vi "菜单-编译.vi"(8 "error in (no error)":errorcluster caption="错误输入（无错误）", 11 "程序响应 输入":refnum<class "程序响应.lvclass">) -> (0 "error out":errorcluster caption="错误输出", 3 "程序响应 输出":refnum<class "程序响应.lvclass">)   [LabVIEW 2020, in "程序响应.lvlib" / "程序响应.lvclass"]
uses:
  D:/SuperPython-master/ScintillaNET.dll
  ScintillaNET.dll
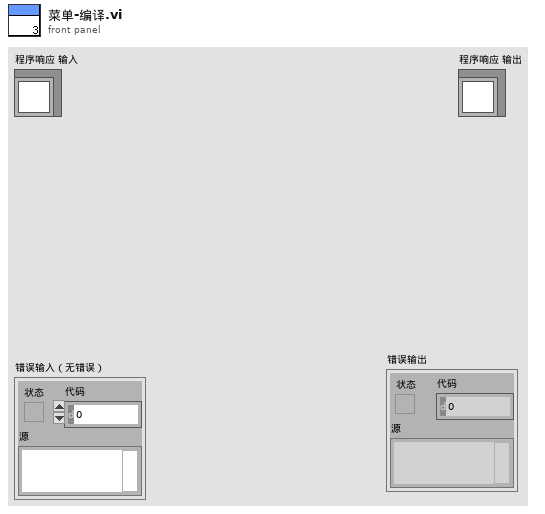
[diagram p1: front panel]
types:
  T1 = enum16{"open", "replace", "create", "open or create", "replace or create", "replace or create with confirmation"}
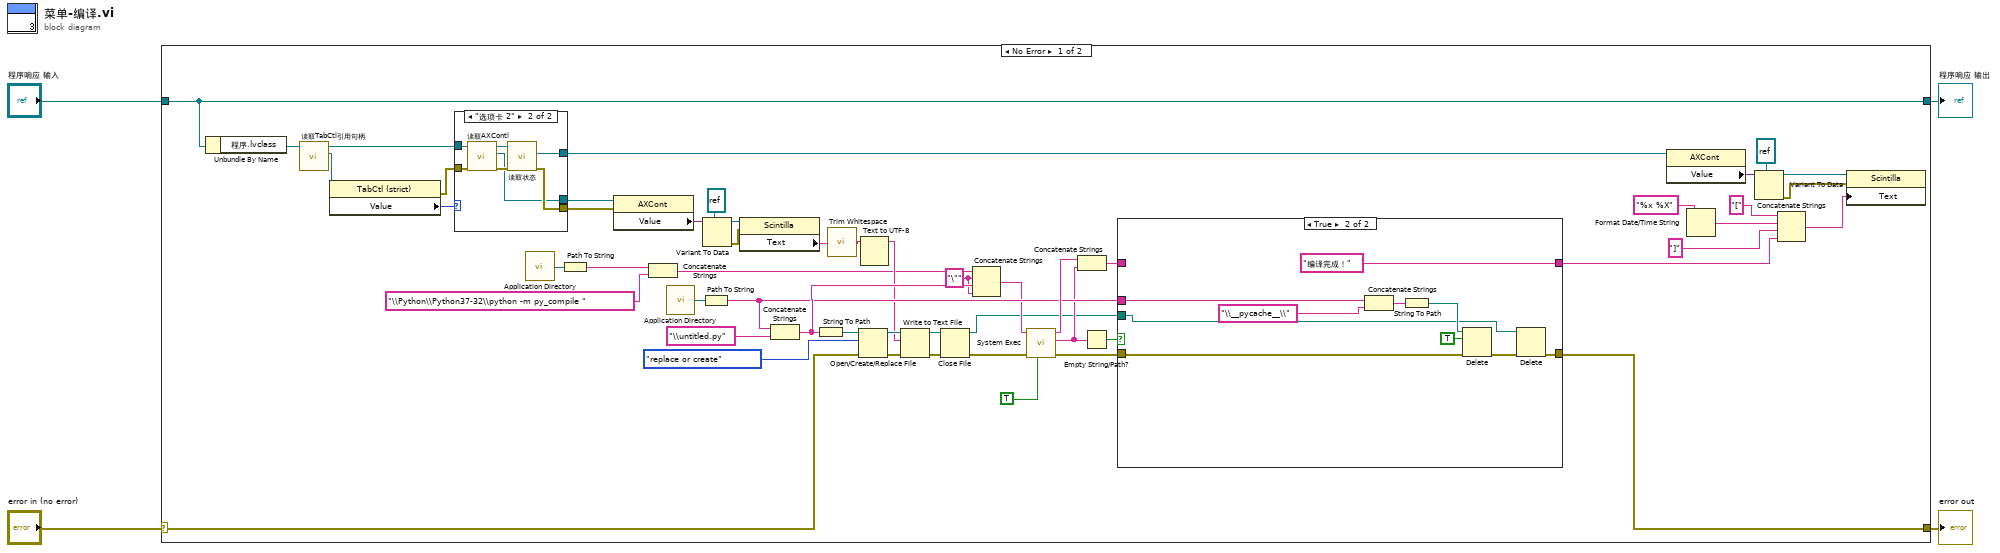
[diagram p0: block diagram]
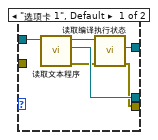
[diagram p2: hidden frame]
diagram:
  n1 = case shown="No Error" "error in (no error)" {
    selector: "error in (no error)" -> [w42 w83]
    tunnel: [w41 w83] -> w3
    tunnel: [w44 w82] -> w1
    tunnel: "程序响应 输入" -> [w44 w82]
    frame No Error {
      w11 = "\"" ("字符串")
      n2 = Unbundle By Name(w44) -> ("程序.lvclass"=w16:refnum<class "程序.lvclass">)
      n3 = call-dynamic "读取TabCtl引用句柄.vi"("程序输入"=w16) -> ("TabCtl引用句柄"=w15:refnum<vi>, "程序输出"=w12:refnum<class "程序.lvclass">)  [unwired: 8 in, 1 out]
      n4 = property class="TabCtl (strict)"(reference=w15) -> (error out=w13:errorcluster, "Value"=w14:enum32{"选项卡 1", "选项卡 2"})  [unwired: 1 in, 1 out]
      n5 = case shown="\"选项卡 2\"" w14 {
        tunnel: [w61 w63] -> w25
        tunnel: [w57 w64] -> w23
        tunnel: [w60 w65] -> w18
        tunnel: w12 -> [w59 w69]
        tunnel: w13 -> [_ w66]
        frame "选项卡 1", Default {
          n6 = call-dynamic "读取文本程序.vi"("程序输入"=w59) -> ("error out"=w58:errorcluster, "文本程序"=w61:refnum<vi>, "程序输出"=w62:refnum<class "程序.lvclass">)  [unwired: 8 in]
          n7 = call-dynamic "读取编译执行状态.vi"("error in (no error)"=w58, "程序输入"=w62) -> ("error out"=w57:errorcluster, "编译执行状态"=w60:refnum<vi>)  [unwired: 7 in, 1 out]
        }
        frame "选项卡 2" {
          n8 = call-dynamic "读取AXContl.vi"("error in (no error)"=w66, "程序输入"=w69) -> ("error out"=w67:errorcluster, "AXContl"=w63:refnum<vi>, "程序输出"=w68:refnum<class "程序.lvclass">)  [unwired: 7 in]
          n9 = call-dynamic "读取状态.vi"("error in (no error)"=w67, "程序输入"=w68) -> ("error out"=w64:errorcluster, "状态"=w65:refnum<vi>)  [unwired: 7 in, 1 out]
        }
      }
      n10 = call <vilib>:"Application Directory.vi"() -> ("Application Directory"=w10:path)
      n11 = Path To String(path=w10) -> (string=w9:string)
      n12 = property class="AXCont"(reference=w25, error in=w23) -> ("Value"=w24:variant)  [unwired: 2 out]
      n13 = Concatenate Strings(w9, "\\Python\\Python37-32\\python -m py_compile " ("字符串")) -> (w7:string)
      n14 = call <vilib>:"Application Directory.vi"() -> ("Application Directory"=w56:path)
      n15 = Path To String(path=w56) -> (string=w40:string)
      n16 = Variant To Data(type=refnum<k24> refnum ("文本编辑"), Variant=w24) -> (data=w27:refnum<k24>, error out=w28:errorcluster)  [unwired: 1 in]
      n17 = property class="Scintilla"(reference=w27, error in=w28) -> ("Text"=w26:string)  [unwired: 2 out]
      n18 = Concatenate Strings(w40, "\\untitled.py" ("字符串")) -> (w47:string)
      n19 = String To Path(string=w47) -> (path=w54:path)
      n20 = call <vilib>:"Trim Whitespace.vi"("string"=w26) -> ("trimmed string"=w31:string)  [unwired: 1 in]
      n21 = Open/Create/Replace File(file path (use dialog)=w54, error in=w42, operation (0:open)=T1."replace or create" ("操作(0:open)")) -> (refnum out=w53:refnum<file>, error out=w52:errorcluster)  [unwired: 3 in, 1 out]
      n22 = Text to UTF-8 ("文本至UTF-8转换")(11:w31) -> (3:w30:string)  [unwired: 2 in, 1 out]
      n23 = Write to Text File(file (use dialog)=w53, text=w30, error in=w52) -> (refnum out=w51:refnum<file>, error out=w50:errorcluster)  [unwired: 1 in, 1 out]
      n24 = Close File(refnum=w51, error in=w50) -> (path=w5:path, error out=w48:errorcluster)
      n25 = Concatenate Strings(w7, w11, w47, w11) -> (w6:string)
      n26 = call <vilib>:"System Exec.vi"("run minimized? (F)"=TRUE, "error in (no error)"=w48, "command line"=w6) -> ("error out"=w46:errorcluster, "standard error"=w39:string, "standard output"=w45:string)  [unwired: 5 in, 1 out]
      n27 = Concatenate Strings(w45, w39) -> (w37:string)
      n28 = Empty String/Path?(string/path=w39) -> (empty?=w38:bool)
      n29 = case shown="True" w38 {
        tunnel: w46 -> [w71 w81]
        tunnel: [w71 w74] -> w41
        tunnel: w40 -> [_ w80]
        tunnel: w37 -> [w70 _]
        tunnel: [w70 "编译完成！"] -> w32
        tunnel: w5 -> [_ w73]
        frame False {
          # "编译不通过"
        }
        frame True {
          n30 = Concatenate Strings(w80, "\\__pycache__\\" ("字符串")) -> (w78:string)
          n31 = String To Path(string=w78) -> (path=w77:path)
          n32 = Delete(path (use dialog)=w77, entire hierarchy (F)=TRUE ("整个层次结构(F)"), error in=w81) -> (error out=w75:errorcluster)  [unwired: 2 in, 2 out]
          n33 = Delete(path (use dialog)=w73, error in=w75) -> (error out=w74:errorcluster)  [unwired: 3 in, 2 out]
        }
      }
      n34 = property class="AXCont"(reference=w18) -> ("Value"=w19:variant)  [unwired: 1 in, 2 out]
      n35 = Format Date/Time String(time format string (%c)="%x %X" ("时间格式字符串(%c)")) -> (date/time string=w33:string)  [unwired: 2 in]
      n36 = Variant To Data(type=refnum<k24> refnum ("文本编辑"), Variant=w19) -> (data=w20:refnum<k24>, error out=w21:errorcluster)  [unwired: 1 in]
      n37 = Concatenate Strings("[" ("字符串"), w33, "]" ("字符串"), w32) -> (w17:string)
      n38 = property class="Scintilla"(reference=w20, error in=w21, "Text"=w17) -> ()  [unwired: 2 out]
    }
    frame Error {
    }
  }
  "error out" <- w3
  "程序响应 输出" <- w1
